vi "2009.vi"() -> ()   [LabVIEW 2009]
panel:
  out "appended array":dbl[](array[numeric])
  in  "Numeric":dbl
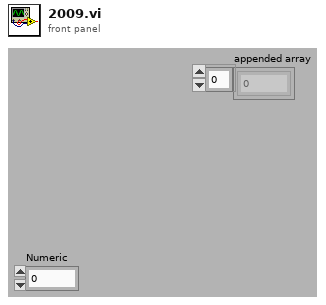
[diagram p1: front panel]
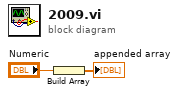
[diagram p0: block diagram]
diagram:
  n1 = Build Array("Numeric") -> (→"appended array":dbl[])
